vi "HapticSPM_write.vi"() -> ()   [LabVIEW 2017]
uses:
  Program Files/National Instruments/LabVIEW 2019/user.lib/Haptic Prog Interface/Haptic Prog Interface.lvlib
  Program Files/National Instruments/LabVIEW 2019/user.lib/Nanonis Prog Interface V5/Nanonis Prog Interface.lvlib
panel:
  out "Force":dbl(slide) scale=0.0..3.0
  out "Force (N)":T1 {"Fz (N)" format="%.1f"; "Fy (N)" format="%.1f"; "Fx (N)" format="%.1f"}
  out "Frame String":string
  in  "Stop":bool
  out "Safe tip":bool
  out "Value":dbl caption="Numeric" format="%#_2p"
  out "Reframed Position (m)":cluster{"x (m)":dbl, "y (m)":dbl, "z (m)":dbl} {"z (m)" format="%.1p"; "y (m)" format="%.1p"; "x (m)" format="%.1p"}
  out "Frame Properties (m)":T2
  in  "Function":string(combo)="0" caption="Combo Box"
  in  "Gain (mm/pm)":dbl=1.0 caption="Numeric" format="%.1g"
  in  "k":dbl=1.0 caption="Numeric" format="%.1g"
  in  "Setpoint":dbl=1e-10 caption="Numeric" format="%.0p"
  in  "Gain":dbl=1.0 caption="Numeric" format="%.1g"
  out "Click Number":dbl caption="Numeric" format="%#_1g"
  in  "Write Z":bool
  in  "Planing Toggle":bool
  in  "Planing Reset":bool
  in  "Save":bool
  out "Surf Loc (m)":dbl
  # "Super Ultra Mega Haptic SPM Controller 3000"
  # "Scan Window"
  # "Signal"
  # "Force"
  # "Planing"
  # "Surface Scale"
  # "Z Write"
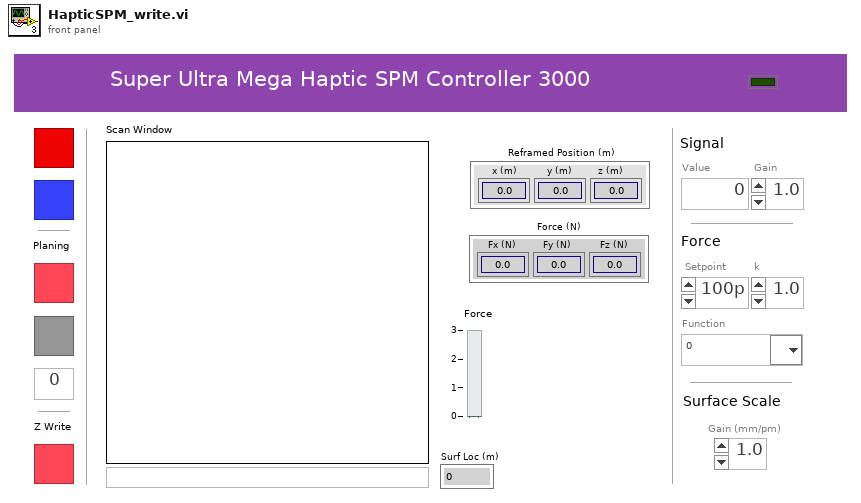
[diagram p1: front panel]
types:
  T1 = cluster{"Fx (N)":dbl, "Fy (N)":dbl, "Fz (N)":dbl}
  T2 = cluster{"Center coordinates (m)":cluster{"Xc":sgl, "Yc":sgl}, "Size (m)":cluster{"Width":sgl, "Height":sgl}}
  T3 = cluster{"kx (N/m)":dbl, "ky (N/m)":dbl, "kz (N/m)":dbl}
  T4 = cluster{"X Drag":bool, "Y Drag":bool, "Z Drag":bool}
  T5 = cluster{"x (mm)":dbl, "y (mm)":dbl, "z (mm)":dbl}
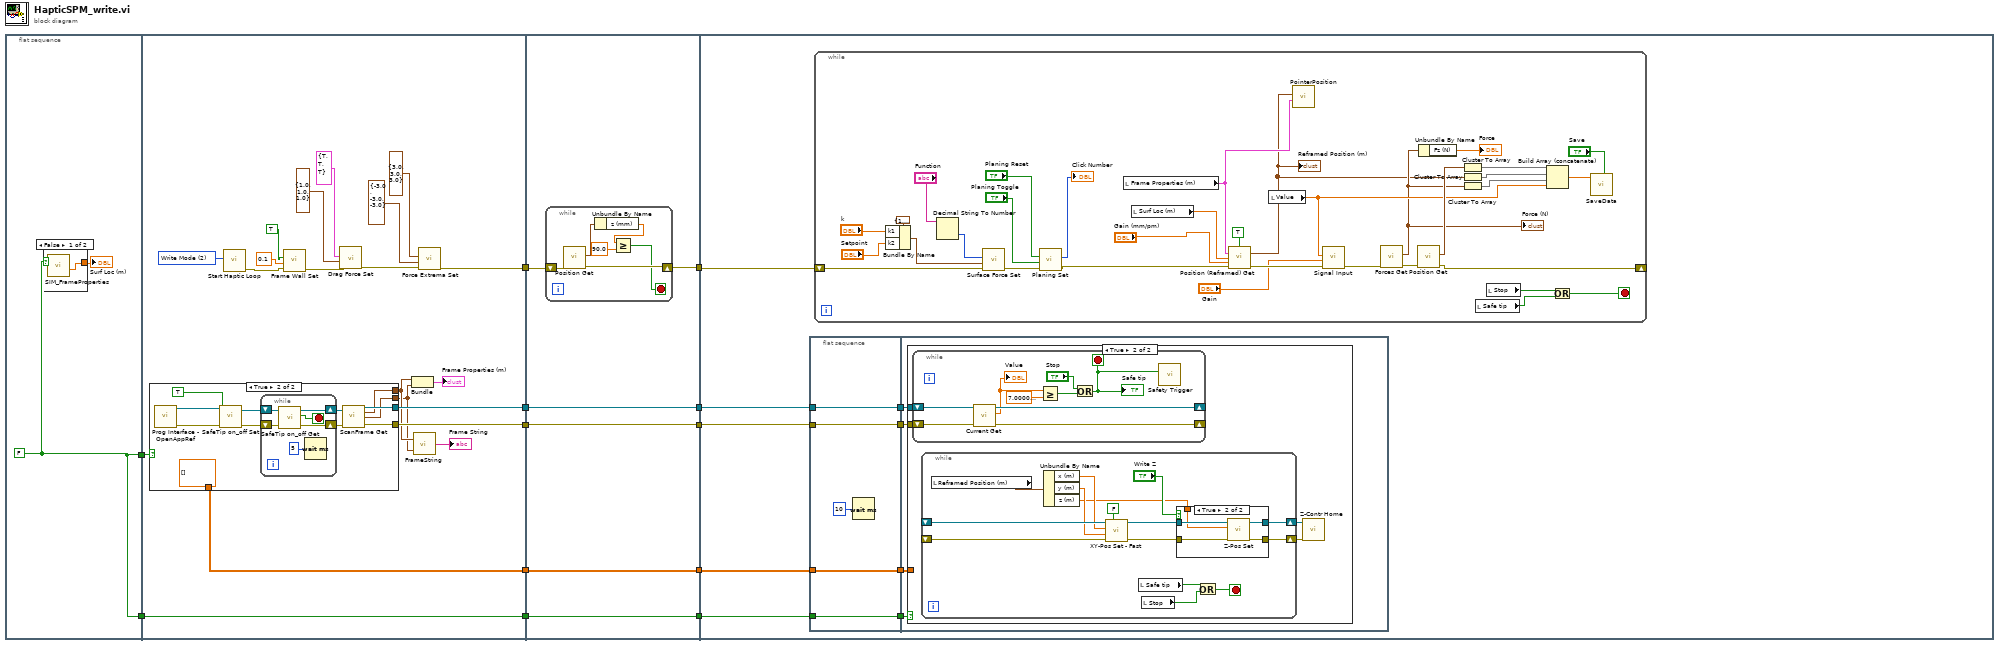
[diagram p0: block diagram]
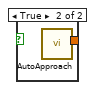
[diagram p2: hidden frame]
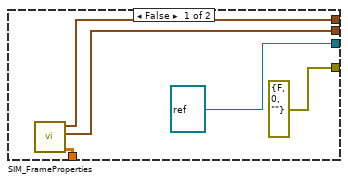
[diagram p3: hidden frame]
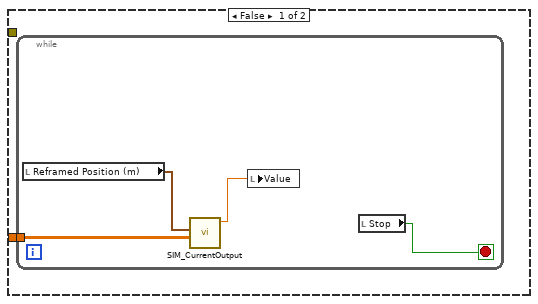
[diagram p4: hidden frame]
diagram:
  n1 = flat-sequence {
    tunnel: [w13] -> w6
    tunnel: [w13] -> w5
    tunnel: [w34] -> w12
    tunnel: [w24] -> w9
    tunnel: [w23] -> w7
    tunnel: w6 -> [w19]
    tunnel: w5 -> [w18]
    tunnel: [w18] -> w4
    tunnel: [w17] -> w1
    tunnel: w12 -> [w65]
    tunnel: [w64] -> w11
    tunnel: [w63] -> w10
    tunnel: w9 -> [w63]
    tunnel: [w62] -> w8
    tunnel: w7 -> [w62]
    tunnel: w4 -> [w61]
    tunnel: [w61] -> w3
    tunnel: [w60] -> w2
    tunnel: w1 -> [w60]
    tunnel: w11 -> [w80]
    tunnel: w10 -> [w78]
    tunnel: w8 -> [w76]
    tunnel: w3 -> [w75]
    tunnel: w2 -> [w72]
    frame #0 {
      w13 = FALSE
      n2 = case shown="False" w13 {
        tunnel: [w15 w16] -> w14
        frame False {
          n3 = call "SIM_FrameProperties.vi"() -> ("Surf Loc (m)"=w15:dbl)  [unwired: 8 in, 3 out]
        }
        frame True {
          n4 = call "AutoApproach.vi"() -> ("Surface Location (m)"=w16:dbl)  [unwired: 11 in]
        }
      }
      "Surf Loc (m)" <- w14
    }
    frame #1 {
      w36 = u16 2 items=["Custom Mode", "Read Mode", "Write Mode"] ("Mode Selection")
      n5 = case shown="True" w19 {
        tunnel: [refnum<vi> refnum ("Application ref out") w46] -> w24
        tunnel: [errorcluster {"status"=FALSE, "code"=0, "source"=""} ("error out") w45] -> w23
        tunnel: [w39 w44] -> w22
        tunnel: [w38 w43] -> w21
        tunnel: [w37 dbl[][] [] ("data")] -> w17
        frame False {
          n6 = call "SIM_FrameProperties.vi"() -> ("data"=w37:dbl[][], "Size (m)"=w38:cluster{"Width":sgl, "Height":sgl}, "Center coordinates (m)"=w39:cluster{"Xc":sgl, "Yc":sgl})  [unwired: 8 in, 1 out]
        }
        frame True {
          n7 = call <userlib>:"Prog Interface - OpenAppRef.vi"() -> ("Error out"=w50:errorcluster, "Application reference"=w49:refnum<vi>)  [unwired: 6 in]
          n8 = call <userlib>:"SafeTip on_off Set.vi"("error in (no error)"=w50, "SafeTip ON/OFF"=TRUE, "Application ref in"=w49) -> ("error out"=w53:errorcluster, "Application ref out"=w52:refnum<vi>)  [unwired: 7 in]
          n9 = while {
            shift-right: [w56] -> w48
            shift-left: w52 -> [w58]
            shift-right: [w55] -> w47
            shift-left: w53 -> [w57]
            stop <- w59 stop-if-true
            n10 = call <userlib>:"SafeTip on_off Get.vi"("error in (no error)"=w57, "Application ref in"=w58) -> ("error out"=w55:errorcluster, "SafeTip on/off status"=w59:bool, "Application ref out"=w56:refnum<vi>)  [unwired: 7 in]
            n11 = Wait (ms)(milliseconds to wait=u32 5) -> ()  [unwired: 1 out]
          }
          n12 = call <userlib>:"ScanFrame Get.vi"("Application ref in"=w48, "error in (no error)"=w47) -> ("Application ref out"=w46:refnum<vi>, "Center coordinates (m)"=w44:cluster{"Xc":sgl, "Yc":sgl}, "Size (m)"=w43:cluster{"Width":sgl, "Height":sgl}, "error out"=w45:errorcluster)  [unwired: 9 in, 1 out]
        }
      }
      n13 = call "Start Haptic Loop.vi"("Mode Selection"=w36) -> ("error out"=w27:errorcluster)  [unwired: 10 in]
      n14 = call "Frame Wall Set.vi"("error in (no error)"=w27, "Wall Stiffness (N/m)"=0.1 ("Wall Stiffness"), "Restrict to Frame"=TRUE) -> ("error out"=w26:errorcluster)  [unwired: 8 in]
      n15 = call "Drag Force Set.vi"("error in (no error)"=w26, "Drag Coefficients (N/m)"=T3 {"kx (N/m)"=1.0, "ky (N/m)"=1.0, "kz (N/m)"=1.0} ("Drag Coefficients"), "Drag Force Toggles"=T4 {"X Drag"=TRUE, "Y Drag"=TRUE, "Z Drag"=TRUE}) -> ("error out"=w35:errorcluster)  [unwired: 8 in]
      n16 = Bundle("Center coordinates (m)"=w22, "Size (m)"=w21) -> (→"Frame Properties (m)":T2)  [unwired: 1 in]
      n17 = call "FrameString.vi"("Size (m)"=w21, "Center coordinates (m)"=w22) -> ("string"=→"Frame String":string)
      n18 = call "Force Extrema Set.vi"("error in (no error)"=w35, "Minimum Force (N)"=T1 {"Fx (N)"=-3.0, "Fy (N)"=-3.0, "Fz (N)"=-3.0} ("Minimum Force"), "Maximum Force (N)"=T1 {"Fx (N)"=3.0, "Fy (N)"=3.0, "Fz (N)"=3.0} ("Maximum Force")) -> ("error out"=w34:errorcluster)  [unwired: 8 in]
    }
    frame #2 {
      n19 = while {
        shift-right: [w70] -> w64
        shift-left: w65 -> [w71]
        stop <- w66 stop-if-true
        n20 = call "Position Get.vi"("error in (no error)"=w71) -> ("error out"=w70:errorcluster, "Position"=w69:T5)  [unwired: 9 in]
        n21 = Unbundle By Name(w69) -> ("z (mm)"=w68:dbl)
        n22 = Greater Or Equal?(x=w68, y=90.0) -> (x >= y?=w66:bool)
      }
    }
    frame #3 {
      n23 = flat-sequence {
        tunnel: [w84] -> w79
        tunnel: w78 -> [w84]
        tunnel: [w83] -> w77
        tunnel: w76 -> [w83]
        tunnel: w75 -> [w82]
        tunnel: [w82] -> w74
        tunnel: [w81] -> w73
        tunnel: w72 -> [w81]
        tunnel: w79 -> [w89]
        tunnel: w77 -> [w88]
        tunnel: w74 -> [w87]
        tunnel: w73 -> [w86]
        frame #0 {
          n24 = Wait (ms)(milliseconds to wait=u32 10) -> ()  [unwired: 1 out]
        }
        frame #1 {
          n25 = case shown="True" w87 {
            tunnel: w89 -> [_ w98]
            tunnel: w88 -> [_ w97]
            tunnel: w86 -> [w90 _]
            frame False {
              n26 = while {
                tunnel: w90 -> [w94]
                stop <- w91 stop-if-true
                n27 = local read "Reframed Position (m)"() -> (w92:cluster{"x (m)":dbl, "y (m)":dbl, "z (m)":dbl})
                n28 = call "SIM_CurrentOutput.vi"("array"=w94, 10:w92) -> ("Current Out (A)"=w93:dbl)  [unwired: 8 in, 1 out]
                n29 = local write "Value"(w93) -> ()
                n30 = local read "Stop"() -> (w91:bool)
              }
            }
            frame True {
              n31 = while {
                shift-right: [w105] -> _
                shift-left: w98 -> [w107]
                shift-right: [w104] -> _
                shift-left: w97 -> [w106]
                stop <- w99 stop-if-true
                n32 = call <userlib>:"Current Get.vi"("Error in (no error)"=w106, "Application ref in"=w107) -> ("Error out"=w104:errorcluster, "Current (A)"=w103:sgl, "Application ref out"=w105:refnum<vi>)  [unwired: 5 in]
                "Value" <- w103
                n33 = Greater Or Equal?(x=w103, y=sgl 7e-10) -> (x >= y?=w101:bool)
                n34 = Or(x="Stop", y=w101) -> (x .or. y?=w99:bool)
                "Safe tip" <- w99
                n35 = call "Safety Trigger.vi"("Safety Trigger"=w99) -> ()  [unwired: 9 in, 2 out]
              }
              n36 = while {
                shift-right: [w115] -> w96
                shift-left: _ -> [w121]
                shift-right: [w113] -> w95
                shift-left: _ -> [w122]
                stop <- w108 stop-if-true
                n37 = local read "Reframed Position (m)"() -> (w120:cluster{"x (m)":dbl, "y (m)":dbl, "z (m)":dbl})
                n38 = Unbundle By Name(w120) -> ("x (m)"=w119:dbl, "y (m)"=w118:dbl, "z (m)"=w111:dbl)
                n39 = call <userlib>:"XY-Pos Set - Fast.vi"("Wait end-of-motion (T=True)"=FALSE, "error in (no error)"=w122, "Y (m)"=w118, "X (m)"=w119, "Application ref in"=w121) -> ("error out"=w112:errorcluster, "Application ref out"=w114:refnum<vi>)  [unwired: 4 in]
                n40 = local read "Safe tip"() -> (w110:bool)
                n41 = local read "Stop"() -> (w109:bool)
                n42 = case shown="True" "Write Z" {
                  tunnel: [w124 w127] -> w115
                  tunnel: w114 -> [w124 w129]
                  tunnel: [w123 w126] -> w113
                  tunnel: w112 -> [w123 w128]
                  tunnel: w111 -> [_ w125]
                  frame False {
                  }
                  frame True {
                    n43 = call <userlib>:"Z-Pos Set.vi"("error in (no error)"=w128, "Z position (m)"=w125, "Application ref in"=w129) -> ("error out"=w126:errorcluster, "Application ref out"=w127:refnum<vi>)  [unwired: 7 in]
                  }
                }
                n44 = Or(x=w110, y=w109) -> (x .or. y?=w108:bool)
              }
              n45 = call <userlib>:"Z-Contr Home.vi"("Error in (no error)"=w95, "Application ref in"=w96) -> ()  [unwired: 8 in, 2 out]
            }
          }
        }
      }
      n46 = while {
        shift-right: [w156] -> _
        shift-left: w80 -> [w163]
        stop <- w134 stop-if-true
        n47 = Bundle By Name(cluster=cluster{"k1":dbl, "k2":dbl, "k3":dbl, "k4":dbl} {"k1"=1.0, "k2"=1.0, "k3"=1.0, "k4"=1.0} ("Force Constants"), "k1"="k", "k2"="Setpoint") -> (w149:cluster{"k1":dbl, "k2":dbl, "k3":dbl, "k4":dbl})
        n48 = Decimal String To Number(string="Function") -> (number=w146:i32)  [unwired: 2 in, 1 out]
        n49 = call "Surface Force Set.vi"("error in (no error)"=w163, "Force Constants"=w149, "Force Settings"=w146) -> ("error out"=w162:errorcluster)  [unwired: 8 in]
        n50 = call "Planing Set.vi"("error in (no error)"=w162, "Planing"="Planing Toggle", "Reset"="Planing Reset") -> ("error out"=w152:errorcluster, "Number of Clicks"=→"Click Number":i8)  [unwired: 7 in]
        n51 = local read "Frame Properties (m)"() -> (w132:T2)
        n52 = local read "Surf Loc (m)"() -> (w160:dbl)
        n53 = call "Position (Reframed) Get.vi"("Z Rescaling"=TRUE, "Frame Properties (m)"=w132, "Surface Location (m)"=w160, "Scaling (mm per pm)"="Gain (mm/pm)", "error in (no error)"=w152) -> ("Reframed Position (m)"=w131:cluster{"x (m)":dbl, "y (m)":dbl, "z (m)":dbl}, "error out"=w158:errorcluster)  [unwired: 9 in]
        "Reframed Position (m)" <- w131
        n54 = local read "Value"() -> (w139:dbl)
        n55 = call "PointerPosition.vi"("Frame Properties (m)"=w132, "Reframed Position (m)"=w131) -> ()  [unwired: 8 in, 2 out]
        n56 = call "Signal Input.vi"("error in (no error)"=w158, "Gain"="Gain", "Signal"=w139) -> ("error out"=w159:errorcluster)  [unwired: 8 in]
        n57 = call "Forces Get.vi"("error in (no error)"=w159) -> ("error out"=w157:errorcluster, "Force (N)"=w133:T1)  [unwired: 9 in]
        "Force (N)" <- w133
        n58 = call "Position Get.vi"("error in (no error)"=w157) -> ("error out"=w156:errorcluster, "Position"=w143:T5)  [unwired: 9 in]
        n59 = Unbundle By Name(w133) -> ("Fz (N)"=→"Force":dbl)
        n60 = Cluster To Array(cluster=w143) -> (array=w142:dbl[])
        n61 = Cluster To Array(cluster=w131) -> (array=w141:dbl[])
        n62 = Cluster To Array(cluster=w133) -> (array=w140:dbl[])
        n63 = local read "Safe tip"() -> (w135:bool)
        n64 = local read "Stop"() -> (w136:bool)
        n65 = Build Array (concatenate)(w142, w141, w140, w139) -> (w138:dbl[])
        n66 = Or(x=w136, y=w135) -> (x .or. y?=w134:bool)
        n67 = call "SaveData.vi"("Save"="Save", "Data"=w138) -> ()  [unwired: 10 in]
      }
    }
  }
